vi "Actor Core.vi"(8 "error in":errorcluster, 11 "Chat Room Controller in":refnum<class "Chat Room Controller.lvclass">) -> (0 "error out":errorcluster, 3 "Actor out":refnum<class "Actor.lvclass">)   [LabVIEW 2018, in "Chat Room Controller.lvlib" / "Chat Room Controller.lvclass"]
doc: "(<B>Filename</B>: Actor Framework.lvlib:Actor.lvclass:Actor Core.vi)\n\nReceives messages to the actor, reacts to them, and initiates any error handling that may shut the actor down.\n\nDescendant classes may override this VI to append parallel tasks for the actor to complete while it handles messages. Overrides use the Call Parent Method node."
uses:
  Chat Room Controller.lvclass
  <vilib>/ActorFramework/Actor/Actor.lvclass
  Chat Room Controller.lvclass/Chat Room Controller.ctl
panel:
  out "Chat Message":string
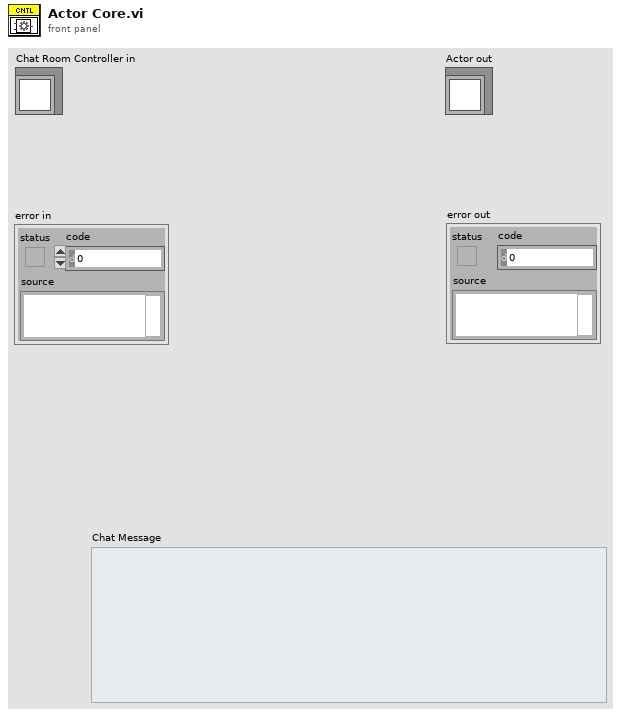
[diagram p1: front panel]
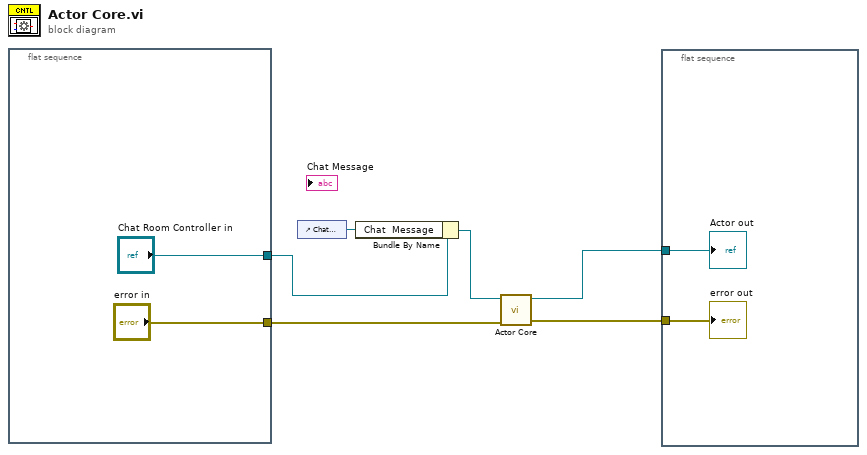
[diagram p0: block diagram]
diagram:
  n1 = flat-sequence {
    tunnel: ["error in"] -> w4
    tunnel: ["Chat Room Controller in"] -> w3
    frame #0 {
    }
  }
  n2 = control-ref of="Chat Message"() -> (w2:refnum<vi>)
  n3 = Bundle By Name(cluster=w3, "Chat  Message"=w2) -> (w1:refnum<class "Chat Room Controller.lvclass">)
  n4 = call-parent "Actor Core.vi"("error in"=w4, "Actor in"=w1) -> ("error out"=w6:errorcluster, "Actor out"=w5:refnum<class "Actor.lvclass">)  [unwired: 8 in]
  n5 = flat-sequence {
    tunnel: w6 -> [w10]
    tunnel: w5 -> [w9]
    frame #0 {
      "error out" <- w10
      "Actor out" <- w9
    }
  }
